vi "Add Section and Channels.vi"(8 "error in (no error)":errorcluster, 11 "Device Item Ref in":T3 format="%.0x") -> (0 "error out":errorcluster, 3 "Item Ref out":T3 format="%.0x")   [LabVIEW 2020, in "PXI-2512 System Explorer.lvlib"]
uses:
  PXI-2512 System Explorer.lvlib
  <vilib>/NI VeriStand/Custom Device API/Custom Device Item Ref.ctl
  <vilib>/NI VeriStand/Custom Device API/Custom Device Channel.ctl
  <vilib>/NI VeriStand/Custom Device API/Custom Device Channel Type.ctl
  Shared/Constants.vi
  <vilib>/NI VeriStand/Custom Device API/Set Item Property (String).vi
  <vilib>/NI VeriStand/Custom Device API/Set Item Property (U16).vi
  <vilib>/NI VeriStand/Custom Device API/Custom Device API.lvlib
  Shared/PXI-2512 Shared.lvlib
panel:
  in  "Channel":T1
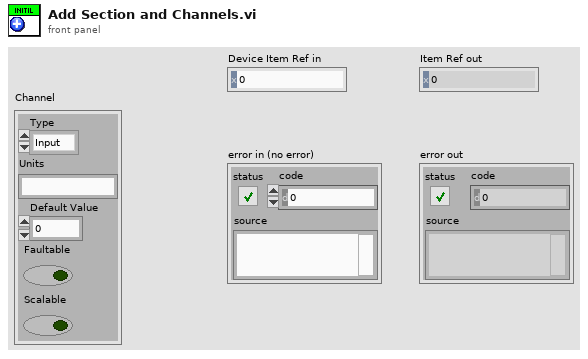
[diagram p1: front panel]
types:
  T1 = typedef "Custom Device API.lvlib/Custom Device Channel.ctl" = cluster{"Type":T2, "Units":string, "Default Value":dbl, "Faultable":bool, "Scalable":bool}
  T2 = typedef "Custom Device API.lvlib/Custom Device Channel Type.ctl" = enum16{"Input", "Output"}
  T3 = typedef "Custom Device API.lvlib/Custom Device Item Ref.ctl" = u64
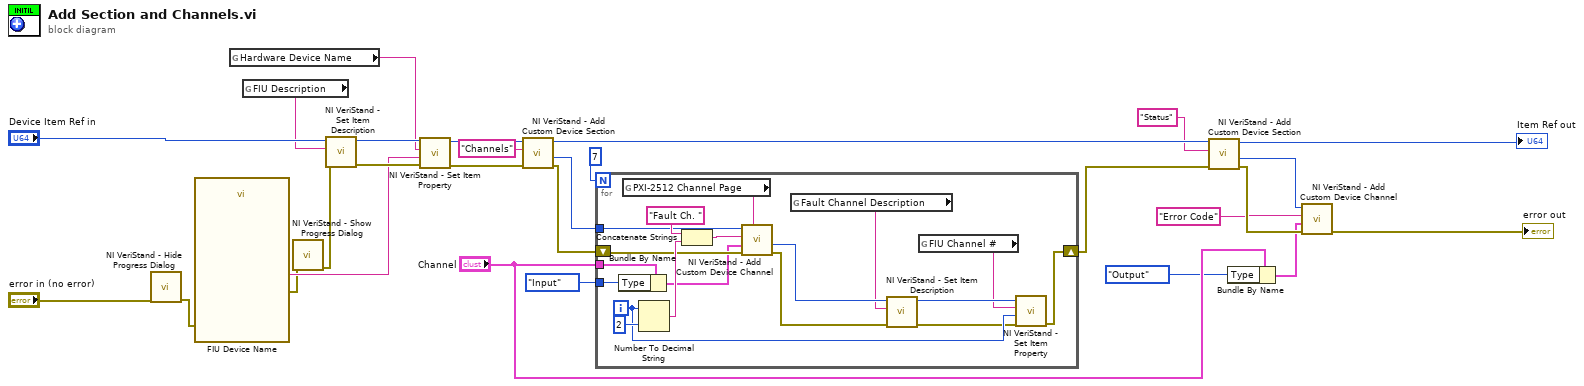
[diagram p0: block diagram]
diagram:
  n1 = call <vilib>:"NI VeriStand - Hide Progress Dialog.vi"("error in (no error)"="error in (no error)") -> ("error out"=w18:errorcluster)  [unwired: 10 in]
  n2 = call "FIU Device Name"("error in (no error)"=w18) -> ("MAX Device Name"=w19:string, "error out"=w17:errorcluster)  [unwired: 16 in, 1 out]
  n3 = global read "Constants.vi" "Hardware Device Name"() -> (w14:string)
  n4 = global read "Constants.vi" "FIU Description"() -> (w13:string)
  n5 = call <vilib>:"NI VeriStand - Show Progress Dialog.vi"("error in (no error)"=w17) -> ("error out"=w16:errorcluster)  [unwired: 10 in]
  n6 = call <vilib>:"NI VeriStand - Set Item Description.vi"("error in (no error)"=w16, "Description"=w13, "Item Ref in"="Device Item Ref in") -> ("error out"=w28:errorcluster, "Item Ref out"=w27:T3)  [unwired: 6 in, 1 out]
  n7 = call-poly <vilib>:"NI VeriStand - Set Item Property.vi"("error in (no error)"=w28, "Value"=w19, "Property Name"=w14, "Item Ref in"=w27) -> ("error out"=w25:errorcluster, "Item Ref out"=w21:T3)  [unwired: 5 in, 1 out]
  n8 = call <vilib>:"NI VeriStand - Add Custom Device Section.vi"("error in (no error)"=w25, "Section Name"="Channels", "Parent Ref in"=w21) -> ("error out"=w23:errorcluster, "Section Ptr"=w20:T3, "Parent Ref out"=w11:T3)  [unwired: 5 in, 1 out]
  n9 = for {
    N: 7 -> [_]
    tunnel: "Channel" -> [w45]
    tunnel: Custom_Device_Channel_Type."Input" ("Type") -> [w41]
    shift-right: [w36] -> w9
    shift-left: w23 -> [w40]
    tunnel: w20 -> [w38]
    i -> [w37]
    n10 = Bundle By Name(cluster=w45, "Type"=w41) -> (w39:T1)
    n11 = global read "Constants.vi" "PXI-2512 Channel Page"() -> (w31:string)
    n12 = Number To Decimal String(number=w37, width (-)=i16 2) -> (decimal integer string=w43:string)
    n13 = Concatenate Strings("Fault Ch. " ("Section Name"), w43) -> (w42:string)
    n14 = call <vilib>:"NI VeriStand - Add Custom Device Channel.vi"("GUID (Default Channel)"=w31, "error in (no error)"=w40, "Channel"=w39, "Channel Name"=w42, "Parent Ref in"=w38) -> ("error out"=w33:errorcluster, "Channel Ref"=w35:T3)  [unwired: 3 in, 2 out]
    n15 = global read "Constants.vi" "Fault Channel Description"() -> (w30:string)
    n16 = call <vilib>:"NI VeriStand - Set Item Description.vi"("error in (no error)"=w33, "Description"=w30, "Item Ref in"=w35) -> ("error out"=w32:errorcluster, "Item Ref out"=w34:T3)  [unwired: 6 in, 1 out]
    n17 = global read "Constants.vi" "FIU Channel #"() -> (w29:string)
    n18 = call-poly <vilib>:"NI VeriStand - Set Item Property.vi"("error in (no error)"=w32, "Value"=w37, "Property Name"=w29, "Item Ref in"=w34) -> ("error out"=w36:errorcluster)  [unwired: 5 in, 2 out]
  }
  n19 = call <vilib>:"NI VeriStand - Add Custom Device Section.vi"("error in (no error)"=w9, "Section Name"="Status" ("Channel Name"), "Parent Ref in"=w11) -> ("error out"=w8:errorcluster, "Section Ptr"=w2:T3, "Parent Ref out"=→"Item Ref out":T3)  [unwired: 5 in, 1 out]
  n20 = Bundle By Name(cluster="Channel", "Type"=Custom_Device_Channel_Type."Output") -> (w3:T1)
  n21 = call <vilib>:"NI VeriStand - Add Custom Device Channel.vi"("error in (no error)"=w8, "Channel"=w3, "Channel Name"="Error Code", "Parent Ref in"=w2) -> ("error out"=→"error out":errorcluster)  [unwired: 4 in, 3 out]
